vi "NIMS_dfd_Convert Band Specs (Group Delay).vi"(8 "W":dbl[](array[numeric]), 9 "Group Delay":dbl[](array[numeric]), 10 "Edges":dbl[](array[numeric]), 11 "F":dbl[](array[numeric])) -> (0 "error out":errorcluster, 2 "band specs":T1[](array[typedef]) {"subband specs"."weight" format="%.2f"})   [LabVIEW 2017, in "NI_DigFilter_MathScript.lvlib"]
uses:
  <vilib>/addons/Digital Filter Design/NI_DigFilter_MathScript.lvlib
  <vilib>/addons/Digital Filter Design/_GroupDelay.llb/dfd_Group Delay_Band Spec.ctl
  <vilib>/addons/Digital Filter Design/_Misc.llb/dfd_Error Handlers (Multiple).vi
  <vilib>/addons/Digital Filter Design/NI_DigFilterLicensed.lvlib
panel:
  # "freq"
  # "group delay"
  # "weight"
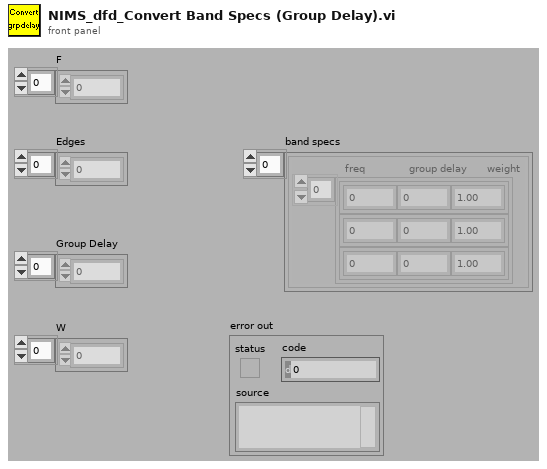
[diagram p1: front panel]
types:
  T1 = typedef "NI_DigFilterLicensed.lvlib/dfd_Group Delay_Band Spec.ctl" = cluster{"subband specs":cluster{"freq":dbl, "group delay":dbl, "weight":dbl}[]}
  T2 = cluster{"Numeric":dbl, "Numeric":dbl, "Numeric":dbl}
  T3 = cluster{cluster{"Numeric":dbl, "Numeric":dbl, "Numeric":dbl}[]}
  T4 = cluster{cluster{"Numeric":dbl, "Numeric":dbl, dbl}[]}
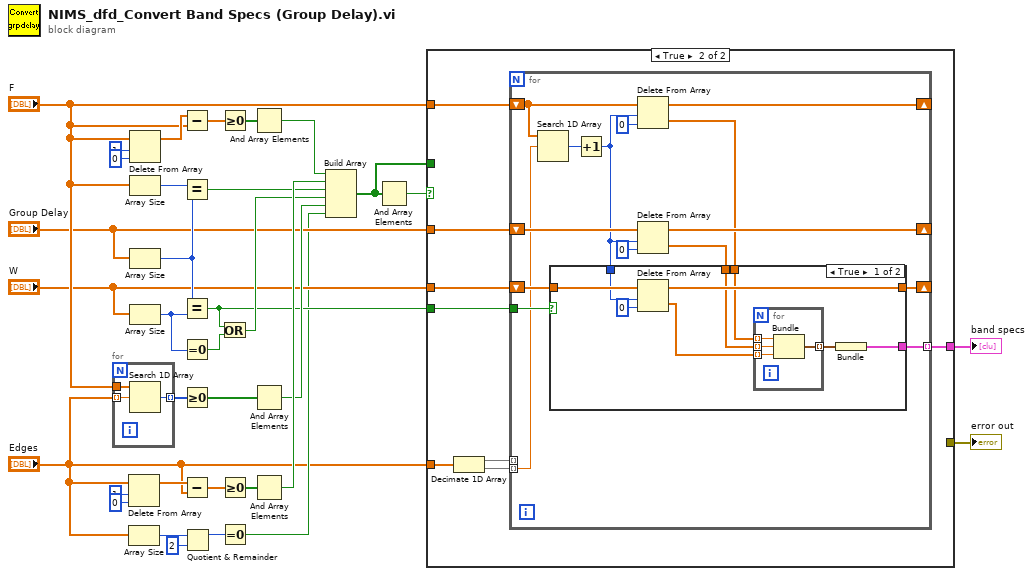
[diagram p0: block diagram]
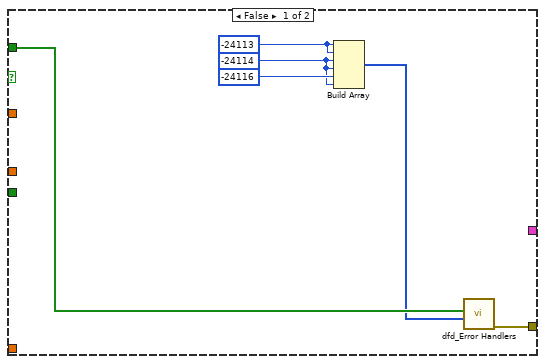
[diagram p2: hidden frame]
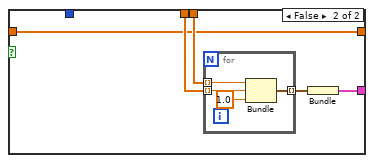
[diagram p3: hidden frame]
diagram:
  n1 = for {
    tunnel: "F" -> [w37]
    tunnel: "Edges" -> [w36] mode=indexing
    tunnel: [w35] -> w19 mode=indexing
    n2 = Search 1D Array(1D array=w37, element=w36) -> (index of element=w35:i32)  [unwired: 1 out]
  }
  n3 = Delete From Array(array="Edges", length=1, index=0) -> (array with subset deleted=w13:dbl[])  [unwired: 1 out]
  n4 = Array Size(array="Edges") -> (size(s)=w7:i32)
  n5 = Delete From Array(array="F", length=1, index=0) -> (array with subset deleted=w32:dbl[])  [unwired: 1 out]
  n6 = Array Size(array="F") -> (size(s)=w26:i32)
  n7 = Array Size(array="Group Delay") -> (size(s)=w25:i32)
  n8 = Array Size(array="W") -> (size(s)=w24:i32)
  n9 = Subtract(x=w32, y="F") -> (x-y=w31:dbl[])
  n10 = Equal?(x=w26, y=w25) -> (x = y?=w21:bool)
  n11 = Equal?(x=w25, y=w24) -> (x = y?=w9:bool)
  n12 = Equal To 0?(x=w24) -> (x = 0?=w10:bool)
  n13 = Greater Or Equal To 0?(x=w19) -> (x >= 0?=w18:bool[])
  n14 = Subtract(x=w13, y="Edges") -> (x-y=w28:dbl[])
  n15 = Quotient & Remainder(x=w7, y=2) -> (x-y*floor(x/y)=w5:i32)  [unwired: 1 out]
  n16 = Greater Or Equal To 0?(x=w31) -> (x >= 0?=w30:bool[])
  n17 = Or(x=w9, y=w10) -> (x .or. y?=w20:bool)
  n18 = Greater Or Equal To 0?(x=w28) -> (x >= 0?=w29:bool[])
  n19 = Equal To 0?(x=w5) -> (x = 0?=w4:bool)
  n20 = And Array Elements(Boolean array=w30) -> (logical AND=w23:bool)
  n21 = And Array Elements(Boolean array=w18) -> (logical AND=w17:bool)
  n22 = And Array Elements(Boolean array=w29) -> (logical AND=w22:bool)
  n23 = Build Array(w23, w22, w21, w20, w17, w4) -> (w1:bool[])
  n24 = And Array Elements(Boolean array=w1) -> (logical AND=w2:bool)
  n25 = case shown="True" w2 {
    tunnel: "F" -> [_ w50]
    tunnel: "Group Delay" -> [_ w49]
    tunnel: "W" -> [_ w48]
    tunnel: "Edges" -> [_ w51]
    tunnel: [_ w47] -> w12
    tunnel: [w43 _] -> w11
    tunnel: w9 -> [_ w46]
    tunnel: w1 -> [w42 _]
    frame False {
      w38 = -24114 ("element")
      w40 = -24113
      n26 = Build Array(w40, w40, w38, w38, -24116 ("element"), w38) -> (w41:i32[])
      n27 = call-poly <vilib>:"dfd_Error Handlers.vi"("error sources"=w41, "condition failed?"=w42) -> ("error out"=w43:errorcluster)  [unwired: 1 in, 8 out]
    }
    frame True {
      n28 = Decimate 1D Array(w51) -> (w45:dbl[], w44:dbl[])
      n29 = for {
        tunnel: w45 -> [_] mode=indexing
        shift-right: [w63] -> _
        shift-left: w50 -> [w66]
        shift-right: [w58] -> _
        shift-left: w49 -> [w61]
        shift-right: [w57] -> _
        shift-left: w48 -> [w60]
        tunnel: [w54] -> w47 mode=indexing
        tunnel: w46 -> [w53]
        tunnel: w44 -> [w52] mode=indexing
        n30 = Search 1D Array(1D array=w66, element=w52) -> (index of element=w64:i32)  [unwired: 1 out]
        n31 = Increment(x=w64) -> (x+1=w59:i32)
        n32 = Delete From Array(array=w66, length=w59, index=0) -> (deleted portion=w56:dbl[], array with subset deleted=w63:dbl[])
        n33 = Delete From Array(array=w61, length=w59, index=0) -> (deleted portion=w55:dbl[], array with subset deleted=w58:dbl[])
        n34 = case shown="True" w53 {
          tunnel: w60 -> [w74 w80]
          tunnel: w59 -> [w73 _]
          tunnel: [w72 w80] -> w57
          tunnel: w56 -> [w71 w84]
          tunnel: w55 -> [w70 w83]
          tunnel: [w67 w81] -> w54
          frame True {
            n35 = Delete From Array(array=w74, length=w73, index=0) -> (deleted portion=w69:dbl[], array with subset deleted=w72:dbl[])
            n36 = for {
              tunnel: w71 -> [w79] mode=indexing
              tunnel: w70 -> [w78] mode=indexing
              tunnel: w69 -> [w77] mode=indexing
              tunnel: [w76] -> w68 mode=indexing
              n37 = Bundle("Numeric"=w79, "Numeric"=w78, "Numeric"=w77) -> (w76:T2)  [unwired: 1 out]
            }
            n38 = Bundle(w68) -> (w67:T3)  [unwired: 1 in]
          }
          frame False {
            n39 = for {
              tunnel: w84 -> [w88] mode=indexing
              tunnel: w83 -> [w87] mode=indexing
              tunnel: [w86] -> w82 mode=indexing
              n40 = Bundle("Numeric"=w88, "Numeric"=w87, 1.0) -> (w86:cluster{"Numeric":dbl, "Numeric":dbl, dbl})  [unwired: 1 out]
            }
            n41 = Bundle(w82) -> (w81:T4)  [unwired: 1 in]
          }
        }
      }
    }
  }
  "band specs" <- w12
  "error out" <- w11
